vi "End Sync Box.vi"(8 "error in (no error)":errorcluster, 11 "SPARC4_GUI in":refnum<class "SPARC4_GUI.lvclass">) -> (0 "error out":errorcluster, 3 "SPARC4_GUI out":refnum<class "SPARC4_GUI.lvclass">)   [LabVIEW 2018, in "SPARC4_GUI.lvclass"]
uses:
  SPARC4_GUI.lvclass
  SPARC4_GUI.lvclass/SPARC4_GUI.ctl
  Sync Box/Sync Box.lvclass
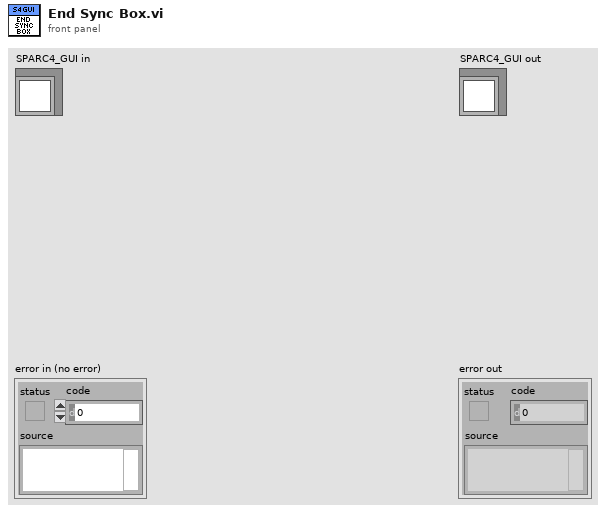
[diagram p1: front panel]
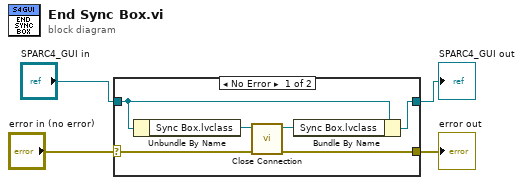
[diagram p0: block diagram]
diagram:
  n1 = case shown="No Error" "error in (no error)" {
    selector: "error in (no error)" -> [w9 w12]
    tunnel: [w10 w12] -> w3
    tunnel: [w6 w11] -> w1
    tunnel: "SPARC4_GUI in" -> [w7 w11]
    frame No Error {
      n2 = Unbundle By Name(w7) -> ("Sync Box.lvclass"=w8:refnum<class "Sync Box.lvclass">)
      n3 = call "Close Connection.vi"("error in (no error)"=w9, "Sync Box in"=w8) -> ("error out"=w10:errorcluster, "Sync Box out"=w5:refnum<class "Sync Box.lvclass">)  [unwired: 8 in]
      n4 = Bundle By Name(cluster=w7, "Sync Box.lvclass"=w5) -> (w6:refnum<class "SPARC4_GUI.lvclass">)
    }
    frame Error {
    }
  }
  "error out" <- w3
  "SPARC4_GUI out" <- w1
